vi "joystick serial.vi"() -> ()   [LabVIEW 2020]
uses:
  <vilib>/Instr/_visa.llb/VISA Configure Serial Port (Instr).vi
panel:
  out "joystick error":errorcluster
  out "v_ang":dbl format="%0.2f"
  out "v_tang":dbl format="%0.2f"
  out "v_norm":dbl format="%0.2f"
  in  "max_v_ang":dbl=3.0 format="%#_13g"
  in  "max_v_norm":dbl=1.0 format="%#_13g"
  in  "max_v_tang":dbl=1.0 format="%#_13g"
  in  "id":u32
  out "Visa return count":u32
  out "String":string
  out "return count":u32
  in  "stop":bool
  out "string":string
  out "error out":errorcluster
  in  "termination char\n(0xA = '\\n' = LF)":u8=10 format="%.0x"
  in  "VISA resource name":refnum<visa-resource-name>
  in  "Serial Settings":T1={"baud rate"=9600, "data bits"=8, "parity"=enum."None", "stop bits"=10, "flow control"=0} {"flow control" items=["None"=0, "XON/XOFF"=1, "RTS/CTS"=2, "DTR/DSR"=4]; "stop bits" items=["1.0"=10, "1.5"=15, "2.0"=20]; "data bits" min=5 max=8 step=1; "baud rate" items=["75"=75, "110"=110, "134"=134, "150"=150, "300"=300, "600"=600, "1200"=1200, "1800"=1800, "2400"=2400, "4800"=4800, "7200"=7200, "9600"=9600, "14400"=14400, "19200"=19200, "28800"=28800, "38400"=38400, "56000"=56000, "57600"=57600, "115200"=115200, "128000"=128000, "230400"=230400]}
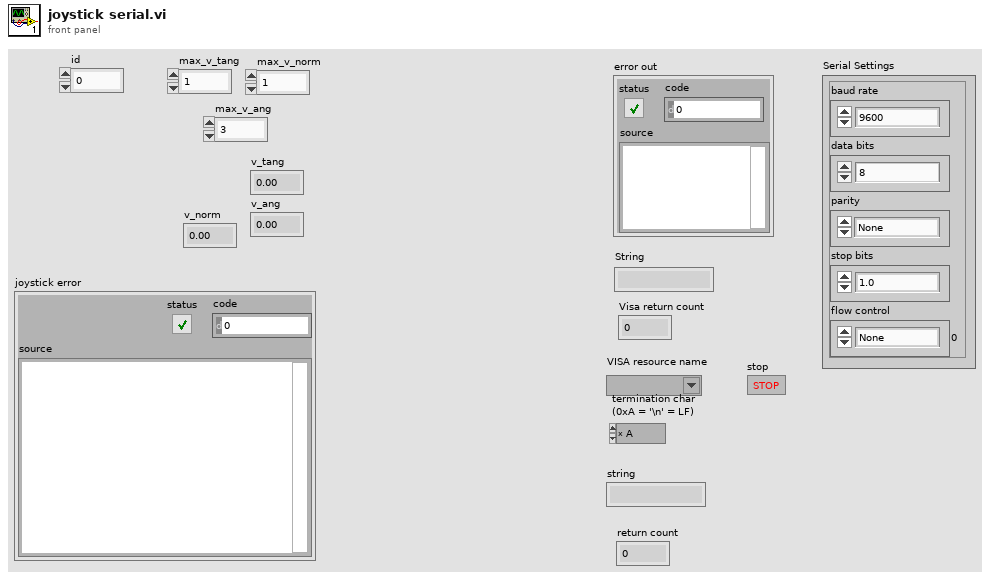
[diagram p1: front panel]
types:
  T1 = cluster{"baud rate":u32, "data bits":u16, "parity":enum16{"None", "Odd", "Even", "Mark", "Space"}, "stop bits":u16, "flow control":u16}
  T2 = typedef "grSim Robot Command.ctl" = cluster{"id":u32, "kickspeedx":sgl, "kickspeedz":sgl, "veltangent":sgl, "velnormal":sgl, "velangular":sgl, "spinner":bool, "wheelspeed":bool, "wheel1":sgl, "wheel2":sgl, "wheel3":sgl, "wheel4":sgl, "kickangle":sgl, "spinner_rpm":sgl}
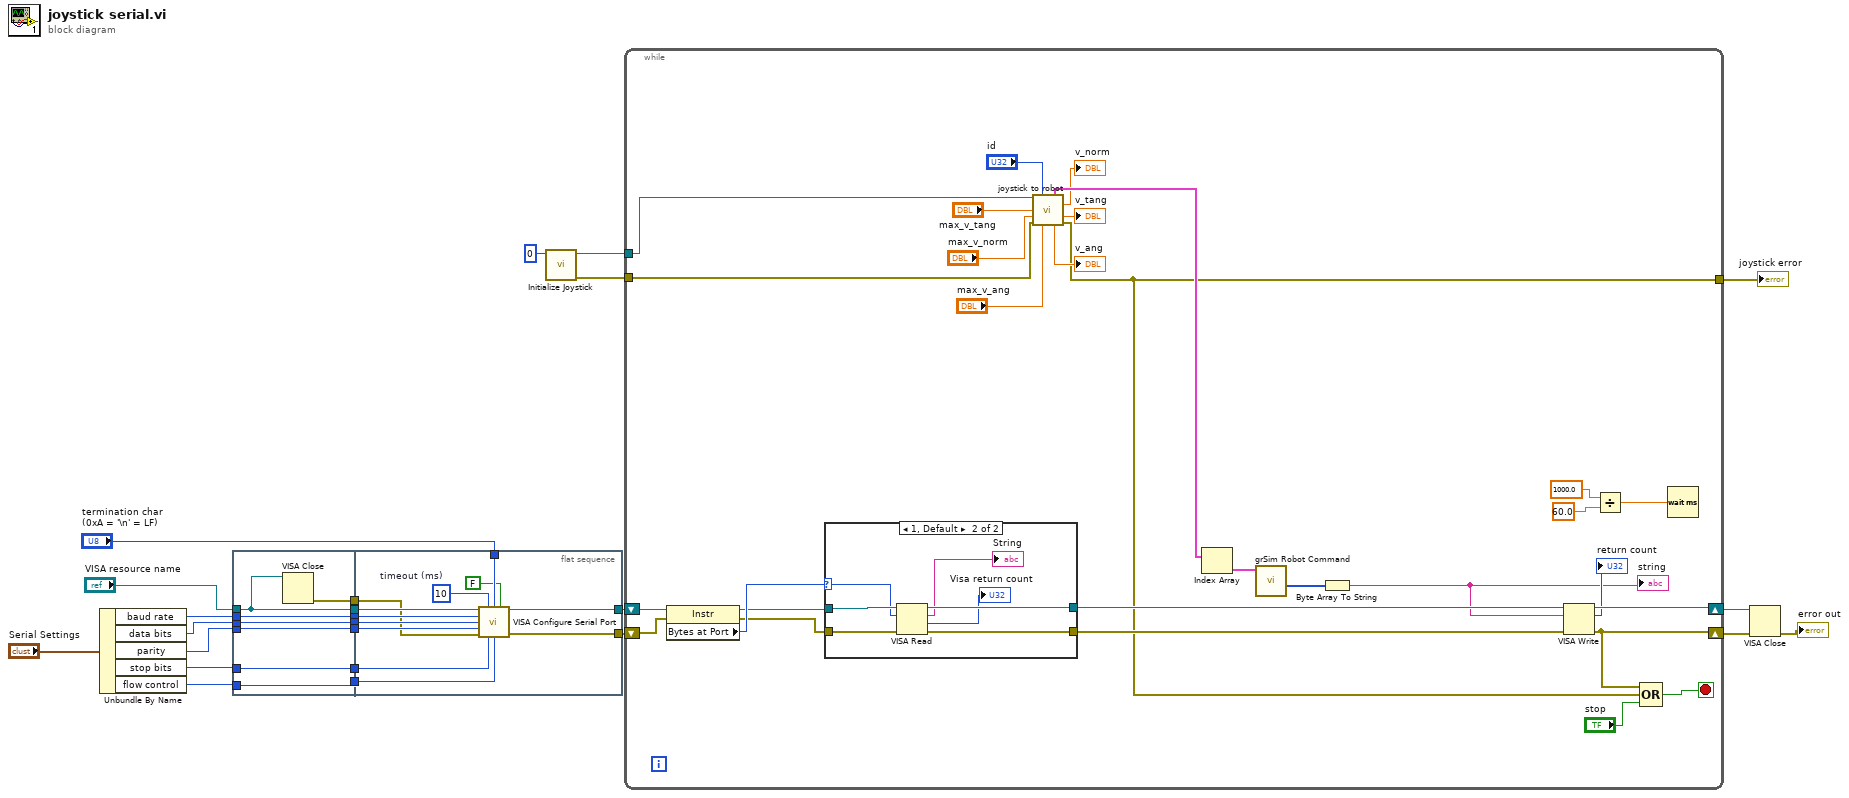
[diagram p0: block diagram]
diagram:
  n1 = Unbundle By Name("Serial Settings") -> ("baud rate"=w23:u32, "data bits"=w22:u16, "parity"=w21:enum16{"None", "Odd", "Even", "Mark", "Space"}, "stop bits"=w20:u16, "flow control"=w19:u16)
  n2 = flat-sequence {
    tunnel: "VISA resource name" -> [w26]
    tunnel: w19 -> [w27]
    tunnel: w20 -> [w28]
    tunnel: w21 -> [w29]
    tunnel: w22 -> [w30]
    tunnel: w23 -> [w31]
    tunnel: [w31] -> w11
    tunnel: [w30] -> w10
    tunnel: [w29] -> w9
    tunnel: [w28] -> w8
    tunnel: [w27] -> w7
    tunnel: [w26] -> w6
    tunnel: [w25] -> w5
    tunnel: "termination char\n(0xA = '\\n' = LF)" -> [w37]
    tunnel: [w35] -> w16
    tunnel: [w34] -> w14
    tunnel: w11 -> [w43]
    tunnel: w10 -> [w42]
    tunnel: w9 -> [w41]
    tunnel: w8 -> [w40]
    tunnel: w7 -> [w39]
    tunnel: w6 -> [w38]
    tunnel: w5 -> [w32]
    frame #0 {
      n3 = VISA Close(VISA resource name=w26) -> (error out=w25:errorcluster)  [unwired: 1 in]
    }
    frame #1 {
      w33 = u32 10  # timeout (ms)
      n4 = call-poly "VISA Configure Serial Port"("VISA resource name"=w38, "timeout (10sec)"=w33, "termination char\n(0xA = '\\n' = LF)"=w37, "Enable Termination\nChar (T)"=FALSE ("Enable Termination\nChar (T)"), "baud rate (9600)"=w43, "data bits (8)"=w42, "parity (0:none)"=w41, "error in (no error)"=w32, "stop bits (10: 1 bit)"=w40, "flow control (0:none)"=w39) -> ("VISA resource name out"=w35:refnum<visa-resource-name>, "error out"=w34:errorcluster)  [unwired: 4 in]
    }
  }
  n5 = call <vilib>:"Initialize Joystick.vi"("device index"=0) -> ("error out"=w2:errorcluster, "device ID"=w3:refnum<k1>)  [unwired: 9 in]
  n6 = while {
    shift-right: [w72] -> w15
    shift-left: w16 -> [w67]
    shift-right: [w70] -> w13
    shift-left: w14 -> [w66]
    tunnel: w3 -> [w56]
    tunnel: w2 -> [w55]
    tunnel: [w44] -> w1
    stop <- w71 stop-if-true
    n7 = property class="Instr"(reference=w67, error in=w66) -> (reference out=w63:refnum<visa-resource-name>, error out=w64:errorcluster, "Bytes at Port"=w65:u32)
    n8 = case shown="1, Default" w65 {
      selector: w65 -> [_ w75]
      tunnel: w64 -> [w73 w81]
      tunnel: [w73 w80] -> w69
      tunnel: w63 -> [w74 w79]
      tunnel: [w74 w78] -> w68
      frame 0 {
      }
      frame 1, Default {
        n9 = VISA Read(VISA resource name=w79, byte count=w75, error in (no error)=w81) -> (VISA resource name out=w78:refnum<visa-resource-name>, read buffer=→"String":string, return count=→"Visa return count":u32, error out=w80:errorcluster)
      }
    }
    n10 = call "joystick to robot.vi"("Refnum in"=w56, "id"="id", "max_v_tang"="max_v_tang", "max_v_norm"="max_v_norm", "error in (no error)"=w55, "max_v_ang"="max_v_ang") -> ("RobotArray"=w54:T2[], "v_norm"=→"v_norm":dbl, "v_tang"=→"v_tang":dbl, "v_ang"=→"v_ang":dbl, "error out"=w44:errorcluster)  [unwired: 4 in, 1 out]
    n11 = Index Array(array=w54) -> (element=w53:T2)  [unwired: 1 in]
    n12 = call "grSim Robot Command.vi"("Robots"=w53) -> ("Array"=w60:u8[])  [unwired: 10 in]
    n13 = Byte Array To String(unsigned byte array=w60) -> (string=w61:string)
    "string" <- w61
    n14 = VISA Write(VISA resource name=w68, write buffer=w61, error in (no error)=w69) -> (VISA resource name out=w72:refnum<visa-resource-name>, return count=→"return count":u32, error out=w70:errorcluster)
    n15 = Divide(x=1000.0, y=60.0) -> (x/y=w58:dbl)
    n16 = Compound Arithmetic op=OR(w70, w44, "stop") -> (w71:bool)
    n17 = Wait (ms)(milliseconds to wait=w58) -> ()  [unwired: 1 out]
  }
  "joystick error" <- w1
  n18 = VISA Close(VISA resource name=w15, error in (no error)=w13) -> (error out=→"error out":errorcluster)
